vi "check if special command.vi"(10 "command":T1) -> (2 "spec CMD":bool)   [LabVIEW 2018, in "LV-0mq-Julia_roundtrip-lib.lvlib"]
uses:
  LV-0mq-Julia_roundtrip-lib.lvlib
  Commands.ctl
panel:
  out "index of element":i32
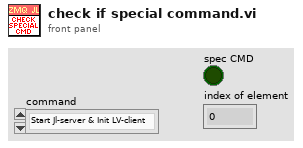
[diagram p1: front panel]
types:
  T1 = typedef "LV-0mq-Julia_roundtrip-lib.lvlib/Commands.ctl" = enum16{"Start Jl-server & Init LV-client", "Send request & Get response ", "Stop Jl-server & Cleanup LV-client", "Cleanup LV-client", "Start Jl-server", "Stop Jl-server", "Init LV-Client", "Cleanup LV-Client", "(not allowed)", "Set LV Client state", "Set Jl Server state", "set ZMQ timeout", "read ZMQ timeout"}
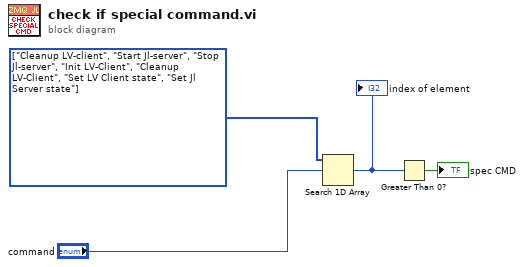
[diagram p0: block diagram]
diagram:
  w4 = T1[] [enum."Cleanup LV-client", enum."Start Jl-server", enum."Stop Jl-server", enum."Init LV-Client", enum."Cleanup LV-Client", enum."Set LV Client state", enum."Set Jl Server state"] items=["Start Jl-server & Init LV-client", "Send request & Get response ", "Stop Jl-server & Cleanup LV-client", "Cleanup LV-client", "Start Jl-server", "Stop Jl-server", "Init LV-Client", "Cleanup LV-Client", "(not allowed)", "Set LV Client state", "Set Jl Server state", "set ZMQ timeout", "read ZMQ timeout"] ("Array")
  n1 = Search 1D Array(1D array=w4, element="command") -> (index of element=w2:i32)  [unwired: 1 in]
  "index of element" <- w2
  n2 = Greater Than 0?(x=w2) -> (x > 0?=→"spec CMD":bool)
